vi "Get Task Rate.vi"(8 "error in":errorcluster, 10 "CD Settings":T1={"CD Task Dependency"=18446744073709551615, "CD Task Dependency Ref"=18446744073709551615, "CD Task Available Wfms"=[], "CD Task Selected Wfms"=[], "Buffer Length (samples)"=0, "Min Enabled"=FALSE, "Max Enabled "=FALSE, "SP Enabled"=FALSE, "RMS Enabled"=FALSE, "Buffer Length (s)"=0.0, "Task Rate"=0.0, "Number of DAQ Chanels"=0} {"CD Task Dependency Ref" format="%.0x"; "CD Task Dependency" format="%.0x"}, 11 "CustomDevice Ref":T2 format="%.0x") -> (0 "error out":errorcluster, 2 "CD Settings out":T1={"CD Task Dependency"=18446744073709551615, "CD Task Dependency Ref"=18446744073709551615, "CD Task Available Wfms"=[], "CD Task Selected Wfms"=[], "Buffer Length (samples)"=0, "Min Enabled"=FALSE, "Max Enabled "=FALSE, "SP Enabled"=FALSE, "RMS Enabled"=FALSE, "Buffer Length (s)"=0.0, "Task Rate"=0.0, "Number of DAQ Chanels"=0} {"CD Task Dependency Ref" format="%.0x"; "CD Task Dependency" format="%.0x"}, 3 "CustomDevice Ref out":T2 format="%.0x")   [LabVIEW 2017, in "Waveform-Processing-Custom-Device System Explorer.lvlib"]
uses:
  Waveform-Processing-Custom-Device System Explorer.lvlib
  <vilib>/NI Veristand/Custom Device API/Custom Device Item Ref.ctl
  Shared/Custom Device Settings.ctl
  NationalInstruments.VeriStand.SystemStorage
  <vilib>/NI Veristand/Custom Device API/Custom Device API.lvlib
  Shared/Waveform-Processing-Custom-Device Shared.lvlib
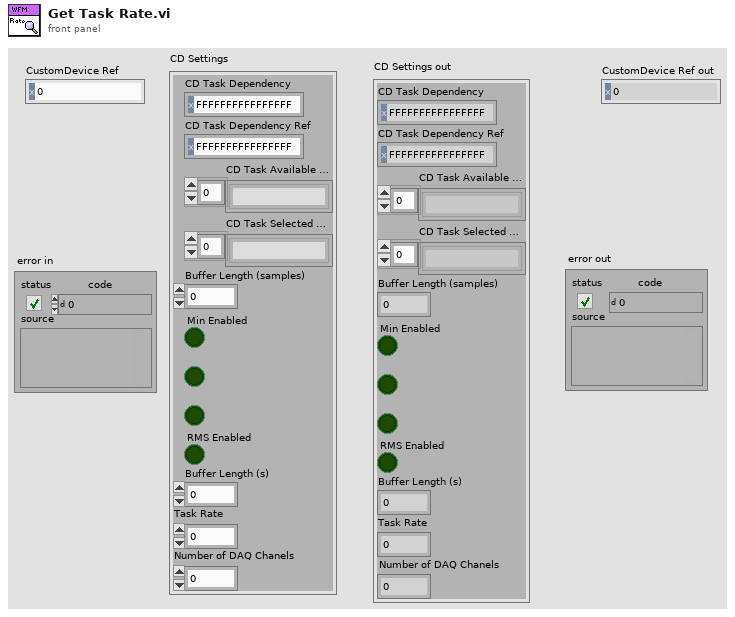
[diagram p1: front panel]
types:
  T1 = typedef "Waveform-Processing-Custom-Device Shared.lvlib/Custom Device Settings.ctl" = cluster{"CD Task Dependency":T2, "CD Task Dependency Ref":T2, "CD Task Available Wfms":string[], "CD Task Selected Wfms":string[], "Buffer Length (samples)":u32, "Min Enabled":bool, "Max Enabled ":bool, "SP Enabled":bool, "RMS Enabled":bool, "Buffer Length (s)":dbl, "Task Rate":dbl, "Number of DAQ Chanels":u32}
  T2 = typedef "Custom Device API.lvlib/Custom Device Item Ref.ctl" = u64
  T3 = typedef "Custom Device API.lvlib/Custom Device Pointer.ctl" = refnum<k24>
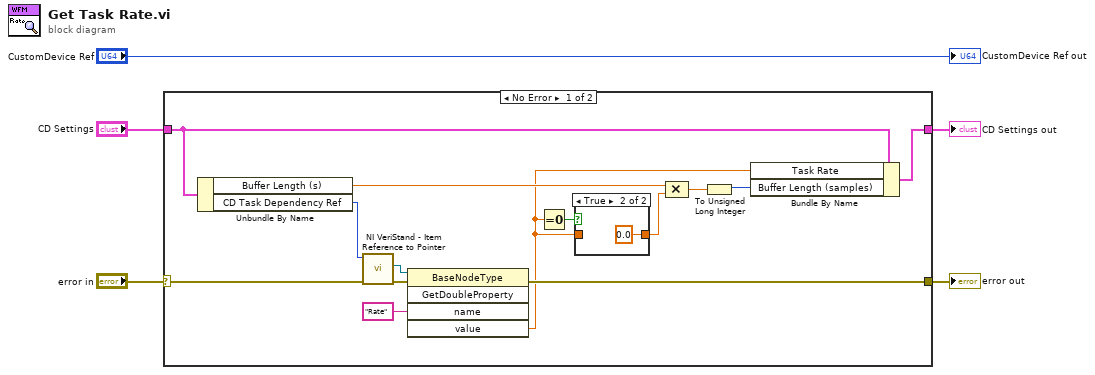
[diagram p0: block diagram]
diagram:
  n1 = case shown="No Error" "error in" {
    selector: "error in" -> [w13 w23]
    tunnel: [w10 w23] -> w4
    tunnel: "CD Settings" -> [w9 w22]
    tunnel: [w6 w22] -> w1
    frame No Error {
      n2 = Unbundle By Name(w9) -> ("Buffer Length (s)"=w11:dbl, "CD Task Dependency Ref"=w17:T2)
      n3 = call <vilib>:"NI VeriStand - Item Reference to Pointer.vi"("error in (no error)"=w13, "Item Ref in"=w17) -> ("error out"=w15:errorcluster, "Node Pointer"=w16:T3)  [unwired: 6 in, 2 out]
      n4 = invoke class="BaseNodeType" method="GetDoubleProperty"(reference=w16, error in=w15, "name"="Rate") -> (error out=w10:errorcluster, "value"=w7:dbl)  [unwired: 2 in, 3 out]
      n5 = Equal To 0?(x=w7) -> (x = 0?=w19:bool)
      n6 = case shown="True" w19 {
        tunnel: [w20 0.0] -> w12
        tunnel: w7 -> [w20 _]
        frame False {
        }
        frame True {
        }
      }
      n7 = Compound Arithmetic op=MULTIPLY(w11, w12) -> (w18:dbl)
      n8 = To Unsigned Long Integer(number=w18) -> (unsigned 32bit integer=w8:u32)
      n9 = Bundle By Name(cluster=w9, "Task Rate"=w7, "Buffer Length (samples)"=w8) -> (w6:T1)
    }
    frame Error {
    }
  }
  "error out" <- w4
  "CD Settings out" <- w1
  "CustomDevice Ref out" <- "CustomDevice Ref"
